vi "find_first_hit.vi"(8 "error in (no error)":errorcluster, 10 "SpaceVector.lvclass":refnum<class "SpaceVector.lvclass">, 11 "RoiCollection in":refnum<class "RoiCollection.lvclass">) -> (0 "error out":errorcluster, 1 "found?":bool, 2 "first hit":refnum<class "RoiGeneric.lvclass">, 3 "RoiCollection out":refnum<class "RoiCollection.lvclass">)   [LabVIEW 2010, in "RoiCollection.lvclass"]
uses:
  RoiCollection.lvclass
  common/classes/SpaceVector/SpaceVector/SpaceVector.lvclass
  RoiGeneric/RoiGeneric.lvclass
  RoiCollection.lvclass/RoiCollection.ctl
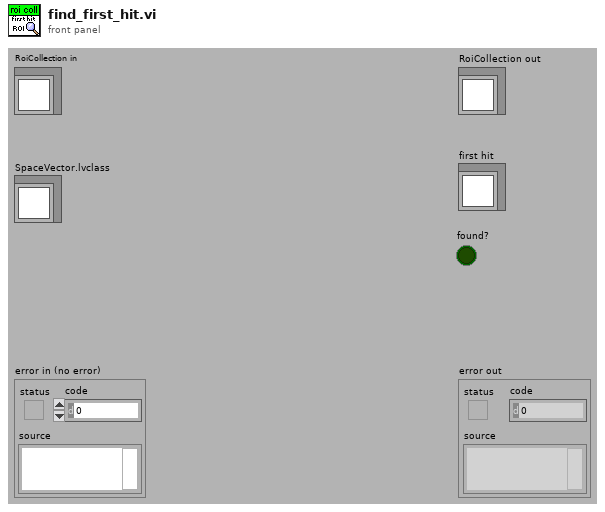
[diagram p1: front panel]
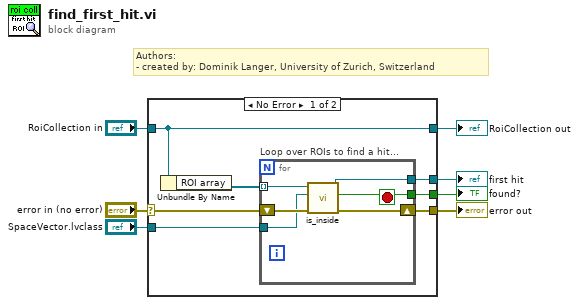
[diagram p0: block diagram]
diagram:
  # "Authors: \n- created by: Dominik Langer, University of Zurich, Switzerland"
  n1 = case shown="No Error" "error in (no error)" {
    selector: "error in (no error)" -> [w8 w22]
    tunnel: [w13 w22] -> w6
    tunnel: [w14 w21] -> w4
    tunnel: "RoiCollection in" -> [w14 w21]
    tunnel: "SpaceVector.lvclass" -> [w9 _]
    tunnel: [w11 _] -> w2
    tunnel: [w10 _] -> w1
    frame No Error {
      n2 = Unbundle By Name(w14) -> ("ROI array"=w12:refnum<class "RoiGeneric.lvclass">[])
      n3 = for "Loop over ROIs to find a hit..." {
        shift-right: [w20] -> w13
        shift-left: w8 -> [w19]
        tunnel: w12 -> [w18] mode=indexing
        tunnel: [w17] -> w11
        tunnel: [w16] -> w10
        tunnel: w9 -> [w15]
        stop <- w16 stop-if-true
        n4 = call-dynamic "is_inside.vi"("error in (no error)"=w19, "SpaceVector.lvclass"=w15, "ROI in"=w18) -> ("error out"=w20:errorcluster, "is inside?"=w16:bool, "ROI out"=w17:refnum<class "RoiGeneric.lvclass">)  [unwired: 6 in]
      }
    }
    frame Error {
    }
  }
  "error out" <- w6
  "RoiCollection out" <- w4
  "first hit" <- w2
  "found?" <- w1
